vi "DeadSnake.vi"(8 "error in (no error)":errorcluster, 11 "Game Data in":T1) -> (0 "error out":errorcluster, 3 "Game Data out":T1)   [LabVIEW 2020]
doc: "Replaces a snake on the board with a dead snake"
uses:
  TypeDef/game-data.ctl
  TypeDef/tiles-key.ctl
  TypeDef/direction.ctl
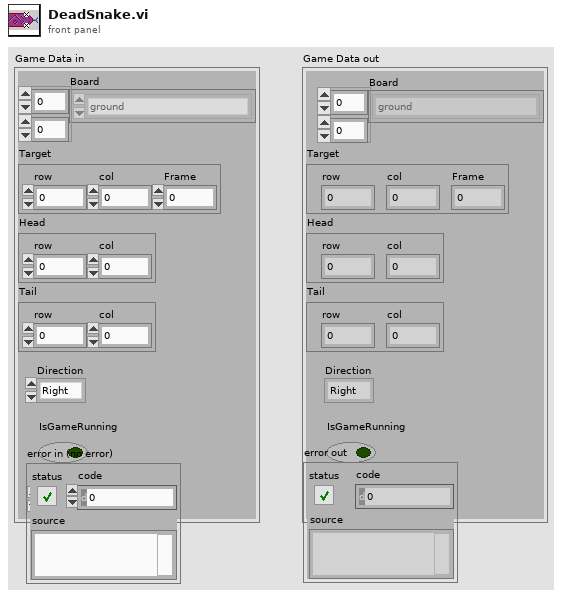
[diagram p1: front panel]
types:
  T1 = typedef "game-data.ctl" = cluster{"Board":T2[][], "Target":cluster{"row":i32, "col":i32, "Frame":i8}, "Head":cluster{"row":i32, "col":i32}, "Tail":cluster{"row":i32, "col":i32}, "Direction":T3, "IsGameRunning":bool, "Points":i32}
  T2 = typedef "tiles-key.ctl" = enum16{"ground", "wall", "head (right)", "head (up)", "head (left)", "head (down)", "L-turn (right-up)", "L-turn (up-left)", "L-turn (left-down)", "L-turn (down-right)", "body (right)", "body (up)", "body (left)", "body (down)", "R-turn (right-down)", "R-turn (up-right)", "R-turn (left-up)", "R-turn (down-left)", "tail (right)", "tail (up)", "tail (left)", "tail (down)", "dead head (right)", "dead head (up)", "dead head (left)", "dead head (down)", "dead L-turn (right-up)", "dead L-turn (up-left)", "dead L-turn (left-down)", "dead L-turn (down-right)", "dead body (right)", "dead body (up)", "dead body (left)", "dead body (down)", "dead R-turn (right-down)", "dead R-turn (up-right)", "dead R-turn (left-up)", "dead R-turn (down-left)", "dead tail (right)", "dead tail (up)", "dead tail (left)", "dead tail (down)", "target red", "target blue", "target yellow", "target green"}
  T3 = typedef "direction.ctl" = enum16{"Right", "Up", "Left", "Down"}
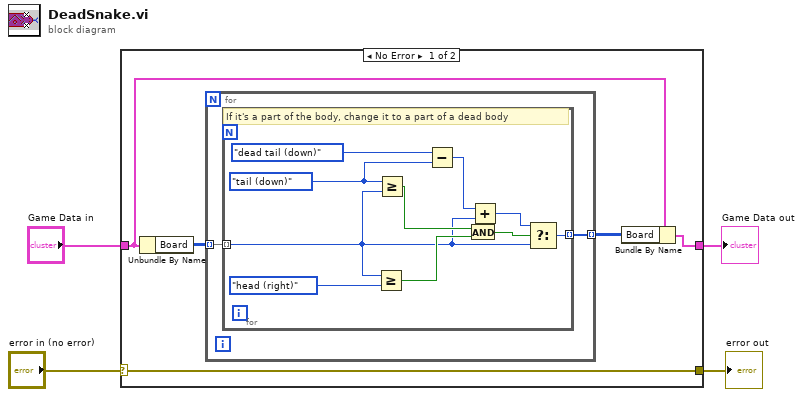
[diagram p0: block diagram]
diagram:
  n1 = case shown="No Error" "error in (no error)" {
    selector: "error in (no error)" -> [w9 w23]
    tunnel: [w9 w23] -> w3
    tunnel: "Game Data in" -> [w7 w22]
    tunnel: [w6 w22] -> w1
    frame No Error {
      n2 = Unbundle By Name(w7) -> ("Board"=w8:T2[][])
      n3 = for {
        tunnel: w8 -> [w11] mode=indexing
        tunnel: [w10] -> w5 mode=indexing
        n4 = for {
          tunnel: w11 -> [w15] mode=indexing
          tunnel: [w14] -> w10 mode=indexing
          w13 = tiles-key."tail (down)" ("x")
          # "If it's a part of the body, change it to a part of a dead body"
          n5 = Greater Or Equal?(x=w15, y=tiles-key."head (right)") -> (x >= y?=w20:bool)
          n6 = Greater Or Equal?(x=w13, y=w15) -> (x >= y?=w21:bool)
          n7 = Subtract(x=tiles-key."dead tail (down)", y=w13) -> (x-y=w17:u16)
          n8 = And(x=w21, y=w20) -> (x .and. y?=w19:bool)
          n9 = Add(x=w17, y=w15) -> (x+y=w16:u16)
          n10 = Select(t=w16, s=w19, f=w15) -> (s? t:f=w14:u16)
        }
      }
      n11 = Bundle By Name(cluster=w7, "Board"=w5) -> (w6:T1)
    }
    frame Error {
    }
  }
  "Game Data out" <- w1
  "error out" <- w3
